vi "EOL Sunshade O'Scope Data.vi"(11 "station names":string[](array[string])) -> ()   [LabVIEW 2018]
uses:
  02.Type Def's/EOL Hall Analog Input Control.ctl
  02.Type Def's/EOL Analog Input Control.ctl
panel:
  out "derecte motor Graph":cluster{"初始x轴值":i32, "△X":i32, sgl[]}(graph)
  in  "station selector":u16(ring) items=["ST40", "ST45"]
  in  "Color Box 16":u32(colorbox)=9567230
  in  "Color Box 15":u32(colorbox)=16711935
  in  "Analog Control 7":T1
  in  "Analog Control 6":T2=enum."ATS"
  in  "Analog Control 5":T1=enum."Sunshade Hall B"
  in  "Analog Control 4":T1
  in  "Analog Control 3":T1=enum."Sunshade Position"
  in  "Analog Control 2":T1=enum."Sunshade Hall B"
  in  "Pause Data Collection":bool
  in  "Color Box 14":u32(colorbox)=15695616
  in  "Color Box 13":u32(colorbox)=1985280
  in  "Analog Control":T1
  in  "Color Box 10":u32(colorbox)=16860
  in  "Color Box 11":u32(colorbox)=16711680
  in  "Color Box 12":u32(colorbox)
  in  "Exit":bool
  # "O'Scope Data Display"
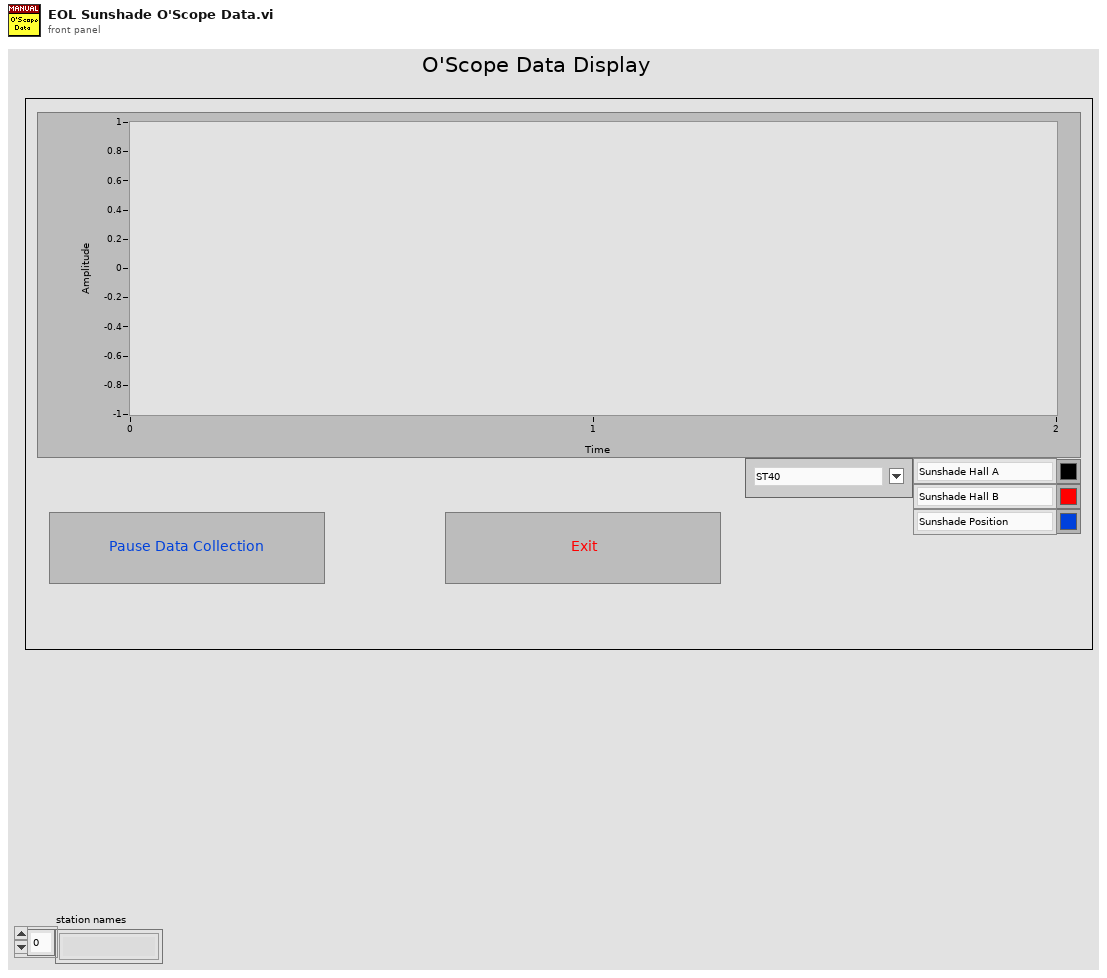
[diagram p1: front panel]
types:
  T1 = typedef "EOL Hall Analog Input Control.ctl" = enum16{"Sunshade Hall A", "Sunshade Hall B", "Sunshade Position"}
  T2 = typedef "EOL Analog Input Control.ctl" = enum16{"SW PS  Volage", "Switch A", "Switch B", "Switch C", "Motor Voltage", "Motor Current", "ATS"}
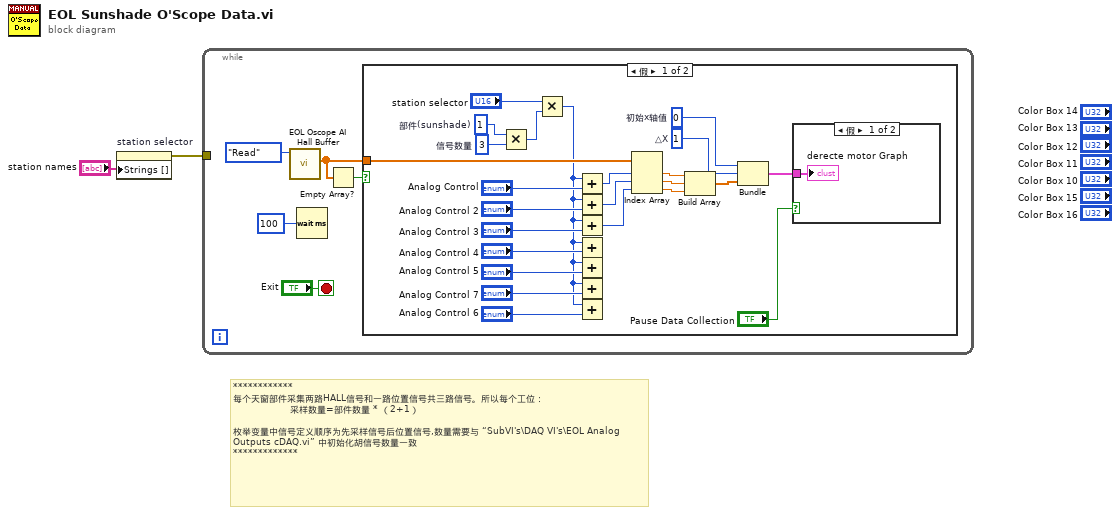
[diagram p0: block diagram]
diagram:
  # "************\n每个天窗部件采集两路HALL信号和一路位置信号共三路信号。所以每个工位：\n                   采样数量=部件数量 * （2+1）\n\n枚举变量中信号定义顺序为先采样信号后位置信号,数量需要与 “SubVI's\\DAQ VI's\\EOL Analog Outputs cDAQ.vi” 中初始化胡信号数量一致 \n*************"
  n1 = property on="station selector" class="Ring (strict)"("Strings []"="station names") -> (error out=w1:errorcluster)  [unwired: 2 in, 1 out]
  n2 = while {
    tunnel: w1 -> [_]
    stop <- "Exit" stop-if-true
    n3 = call "EOL Oscope AI Hall Buffer.vi"("Mode"=enum16{"Initialize", "Read", "Write"}."Read") -> ("Data Read (Single)"=w3:sgl[])  [unwired: 10 in]
    n4 = Wait (ms)(milliseconds to wait=u32 100) -> ()  [unwired: 1 out]
    n5 = Empty Array?(array=w3) -> (empty?=w5:bool)
    n6 = case shown="假" w5 {
      tunnel: w3 -> [w26 _]
      frame False {
        w14 = 1  # △X
        w13 = 0  # 初始x轴值
        w29 = 1  # 部件(sunshade)
        w28 = 3  # 信号数量
        n7 = Multiply(x=w29, y=w28) -> (x*y=w27:i32)
        n8 = Multiply(x="station selector", y=w27) -> (x*y=w17:i32)
        n9 = Add(x=w17, y="Analog Control") -> (x+y=w24:i32)
        n10 = Add(x=w17, y="Analog Control 2") -> (x+y=w16:i32)
        n11 = Add(x=w17, y="Analog Control 3") -> (x+y=w15:i32)
        n12 = Add(x=w17, y="Analog Control 4") -> ()  [unwired: 1 out]
        n13 = Add(x=w17, y="Analog Control 5") -> ()  [unwired: 1 out]
        n14 = Add(x=w17, y="Analog Control 7") -> ()  [unwired: 1 out]
        n15 = Add(x=w17, y="Analog Control 6") -> ()  [unwired: 1 out]
        n16 = Index Array(array=w26, index #1=w24, index #2=w16, index #3=w15) -> (element #1=w12:sgl, element #2=w11:sgl, element #3=w10:sgl)
        n17 = Build Array(w12, w11, w10) -> (w9:sgl[])
        n18 = Bundle("初始x轴值"=w13, "△X"=w14, w9) -> (w8:cluster{"初始x轴值":i32, "△X":i32, sgl[]})  [unwired: 1 in]
        n19 = case shown="假" "Pause Data Collection" {
          tunnel: w8 -> [w32 _]
          frame False {
            "derecte motor Graph" <- w32
          }
          frame True {
          }
        }
      }
      frame True {
      }
    }
  }
